vi "Balance.vi"(8 "file path":path, 9 "Account No.":string, 10 "after match":string) -> (2 "Output":string)   [LabVIEW 2023]
uses:
  <vilib>/Utility/file.llb/Read Delimited Spreadsheet (string).vi
panel:
  # "Output"
  # "Input"
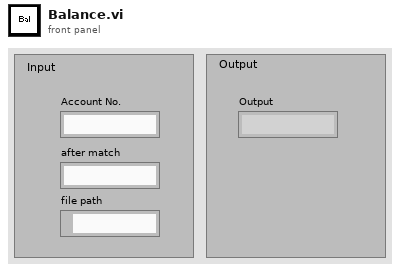
[diagram p1: front panel]
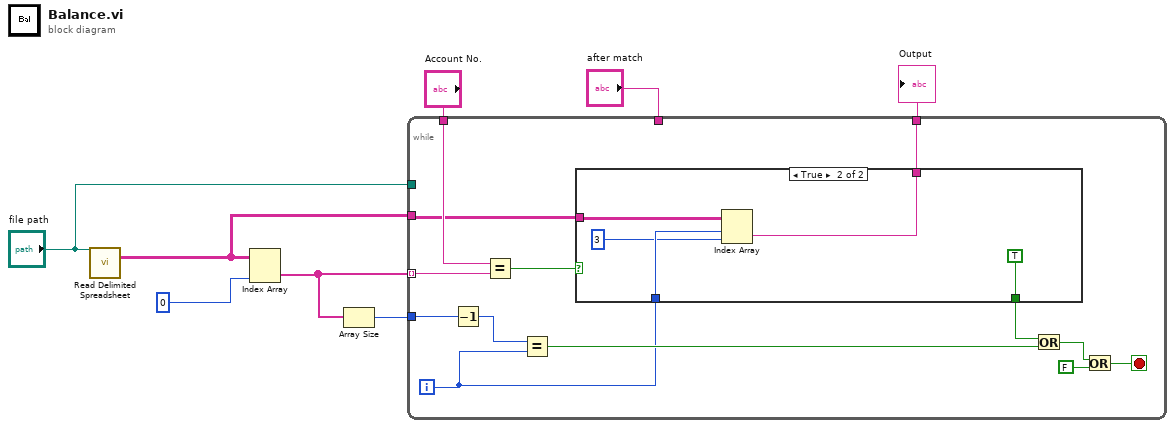
[diagram p0: block diagram]
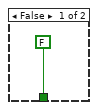
[diagram p2: hidden frame]
diagram:
  n1 = call-poly <vilib>:"Read Delimited Spreadsheet.vi"("file path (dialog if empty)"="file path") -> ("all rows"=w6:string[][])  [unwired: 9 in, 5 out]
  n2 = Index Array "Index Array"(array=w6, index (col)=0 ("index")) -> (element=w7:string[])  [unwired: 1 in]
  n3 = Array Size(array=w7) -> (size(s)=w8:i32)
  n4 = while {
    tunnel: w8 -> [w19]
    tunnel: w7 -> [w17] mode=indexing
    tunnel: w6 -> [w15]
    tunnel: "file path" -> [_]
    tunnel: "Account No." -> [w16]
    tunnel: [w9] -> w2
    tunnel: "after match" -> [_]
    i -> [w10]
    stop <- w21 stop-if-true
    n5 = Decrement(x=w19) -> (x-1=w20:i32)
    n6 = Equal?(x=w16, y=w17) -> (x = y?=w14:bool)
    n7 = Equal?(x=w20, y=w10) -> (x = y?=w12:bool)
    n8 = case shown="True" w14 {
      tunnel: w15 -> [_ w26]
      tunnel: [FALSE TRUE ("x")] -> w11
      tunnel: w10 -> [_ w25]
      tunnel: [_ w23] -> w9
      frame False {
      }
      frame True {
        n9 = Index Array "Index Array"(array=w26, index (row)=w25, index (col)=3 ("disabled index (col)")) -> (element=w23:string)
      }
    }
    n10 = Or(x=w11, y=w12) -> (x .or. y?=w13:bool)
    n11 = Or(x=w13, y=FALSE) -> (x .or. y?=w21:bool)
  }
  "Output" <- w2
